vi "AcqVideoOptCodes.vi"(8 "error in (no error)":errorcluster, 11 "CameraTesting in":refnum<class "CameraTesting.lvclass">) -> (0 "error out":errorcluster, 3 "CameraTesting out":refnum<class "CameraTesting.lvclass">)   [LabVIEW 2020, in "CameraTesting.lvlib" / "CameraTesting.lvclass"]
uses:
  CameraTesting.lvclass
  CameraTesting.lvclass/CameraTesting.ctl
  Camera/ICamera/ICamera/ICamera.lvclass
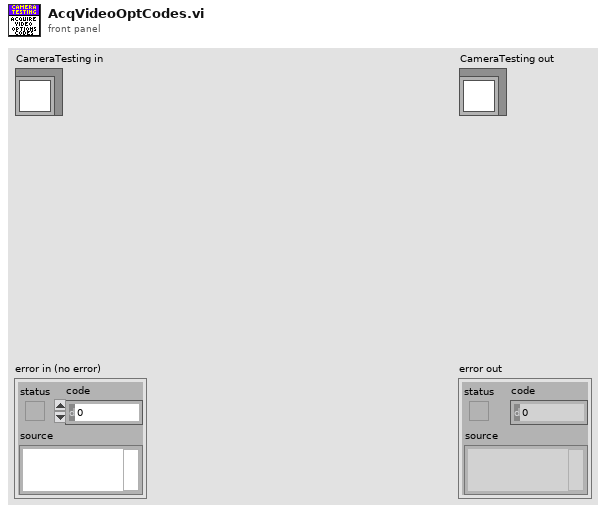
[diagram p1: front panel]
types:
  T1 = typedef "ICameraTesting.lvlib/ICameraTesting.lvclass/VideoOptCodesUpdated.ctl" = refnum<user-event>
  T2 = typedef "ICamera.lvlib/ICamera.lvclass/VideoOptionsCodes.ctl" = cluster{"FrameRateCodesList":cluster{"Description":string, "Code":u8}[], "VideoResolutionCodesList":cluster{"Description":string, "Code":u8}[], "ImageTypeCodesList":cluster{"Description":string, "Code":u8}[]}
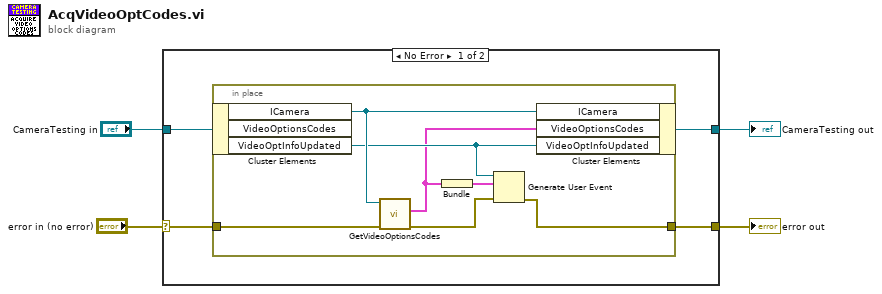
[diagram p0: block diagram]
diagram:
  n1 = case shown="No Error" "error in (no error)" {
    selector: "error in (no error)" -> [w7 w16]
    tunnel: "CameraTesting in" -> [w8 w17]
    tunnel: [w6 w17] -> w2
    tunnel: [w5 w16] -> w1
    frame No Error {
      n2 = in-place {
        in-place-border: w7 -> [w13]
        in-place-border: [w12] -> w5
        n3 = in-place-cluster #1(w8) -> ("ICamera"=w15:refnum<class "ICamera.lvclass">, "VideoOptInfoUpdated"=w14:T1)  [unwired: 1 out]
        n4 = call-dynamic "GetVideoOptionsCodes.vi"("error in (no error)"=w13, "ICamera in"=w15) -> ("error out"=w11:errorcluster, "VideoOptionsCodes"=w10:T2)  [unwired: 7 in, 1 out]
        n5 = Bundle("VideoOptionsCodes"=w10) -> (w9:cluster{"VideoOptionsCodes":T2})  [unwired: 1 in]
        n6 = Generate User Event(user event=w14, event data cluster=w9, error in=w11) -> (error out=w12:errorcluster)  [unwired: 1 in, 1 out]
        n7 = in-place-cluster #1("ICamera"=w15, "VideoOptionsCodes"=w10, "VideoOptInfoUpdated"=w14) -> (w6:refnum<class "CameraTesting.lvclass">)
      }
    }
    frame Error {
    }
  }
  "error out" <- w1
  "CameraTesting out" <- w2
